vi "Post-Run Action.vi"(8 "error in (no error)":errorcluster, 10 "Passed? in":bool, 11 "Project Builder in":refnum<class "Project Builder.lvclass">) -> (0 "error out":errorcluster, 2 "Passed? out":bool, 3 "Project Builder out":refnum<class "Project Builder.lvclass">)   [LabVIEW 2019, in "ProjectBuilder.lvlib" / "Project Builder.lvclass"]
doc: "Override to implement and action at the end of the Build Project.vi.\n\nThe default implementation does nothing."
uses:
  Project Builder.lvclass
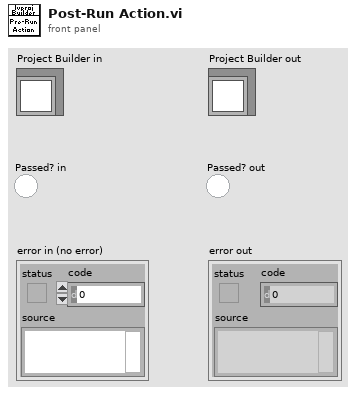
[diagram p1: front panel]
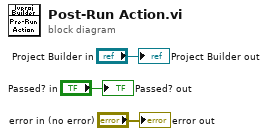
[diagram p0: block diagram]
diagram:
  "error out" <- "error in (no error)"
  "Project Builder out" <- "Project Builder in"
  "Passed? out" <- "Passed? in"
